vi "VITAC Getting Started.vi"   [LabVIEW 2015]
uses:
  <vilib>/Platform/browser.llb/Open URL in Default Browser (string).vi
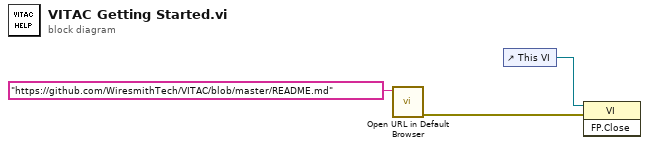
[diagram p0: block diagram]
diagram:
  n1 = call-poly <vilib>:"Open URL in Default Browser.vi"("URL"="https://github.com/WiresmithTech/VITAC/blob/master/README.md") -> ("error out"=w1:errorcluster)  [unwired: 5 in, 1 out]
  n2 = control-ref of="This VI"() -> (w2:refnum<vi>)
  n3 = invoke class="VI" method="FP.Close"(reference=w2, error in=w1) -> ()  [unwired: 1 in, 3 out]
